vi "loading modules message.vi"(8 "error in":errorcluster) -> (0 "error out":errorcluster)   [LabVIEW 2012]
panel:
  out "Boolean":bool=TRUE
  out "String 3":string
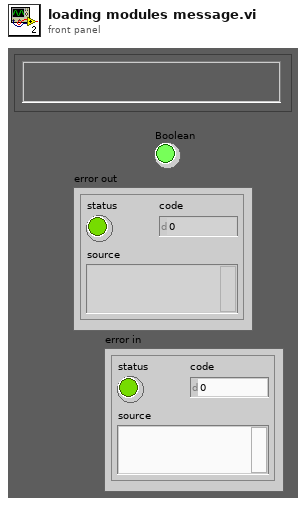
[diagram p1: front panel]
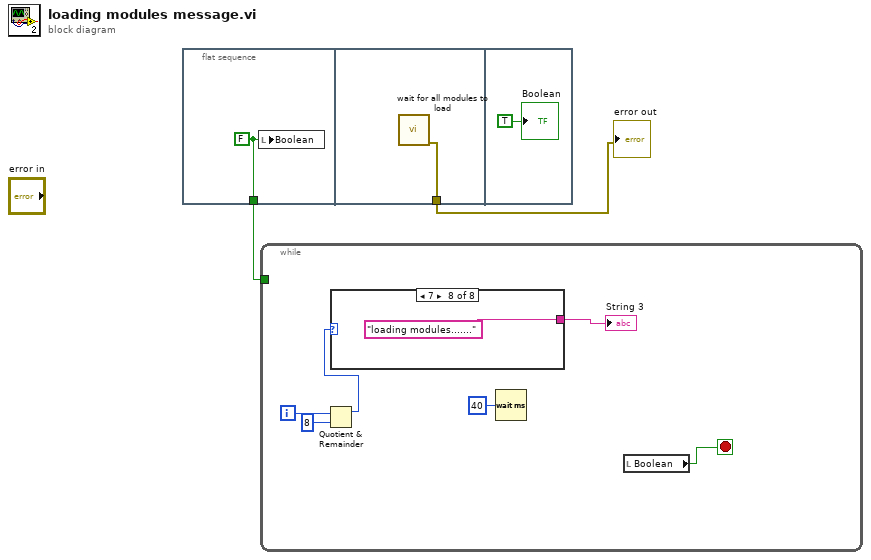
[diagram p0: block diagram]
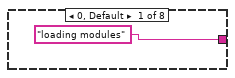
[diagram p2: hidden frame]
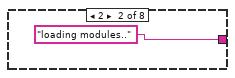
[diagram p3: hidden frame]
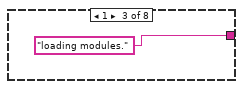
[diagram p4: hidden frame]
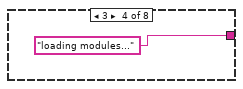
[diagram p5: hidden frame]
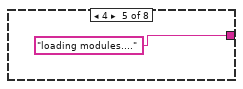
[diagram p6: hidden frame]
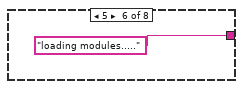
[diagram p7: hidden frame]
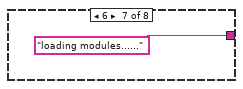
[diagram p8: hidden frame]
diagram:
  n1 = flat-sequence {
    tunnel: [w3] -> w2
    tunnel: [w4] -> w1
    frame #0 {
      w3 = FALSE ("Boolean")
      n2 = local write "Boolean"(w3) -> ()
    }
    frame #1 {
      n3 = call "wait for all modules to load.vi"() -> ("error out"=w4:errorcluster)  [unwired: 11 in]
    }
    frame #2 {
      "Boolean" <- TRUE
    }
  }
  n4 = while {
    tunnel: w2 -> [_]
    i -> [w9]
    stop <- w6 stop-if-true
    n5 = Quotient & Remainder(x=w9, y=8) -> (x-y*floor(x/y)=w7:i32)  [unwired: 1 out]
    n6 = case shown="7" w7 {
      tunnel: ["loading modules" "loading modules.." "loading modules." "loading modules..." "loading modules...." "loading modules....." "loading modules......" "loading modules......."] -> w11
      frame 0, Default {
      }
      frame 2 {
      }
      frame 1 {
      }
      frame 3 {
      }
      frame 4 {
      }
      frame 5 {
      }
      frame 6 {
      }
      frame 7 {
      }
    }
    "String 3" <- w11
    n7 = Wait (ms)(milliseconds to wait=u32 40) -> ()  [unwired: 1 out]
    n8 = local read "Boolean"() -> (w6:bool)
  }
  "error out" <- w1
